vi "User Event AE.vi"(0 "Mode":T3(ring)=enum."Post Event", 1 "Event Name":string, 2 "Event Data":variant, 5 "error in (no error)":errorcluster caption="错误输入（无错误）", 6 "Tag":T1) -> (14 "Event Registration Refnum":T2, 19 "error out":errorcluster caption="错误输出")   [LabVIEW 2013, in "User Event Collection.lvclass"]
uses:
  User Event Collection.lvclass
  <resource>/importtools/Common/Event/Data Type/Event Registeration Refnum.ctl
  Method/Tag.ctl
  <resource>/importtools/Common/Event/NISAST Event.lvclass
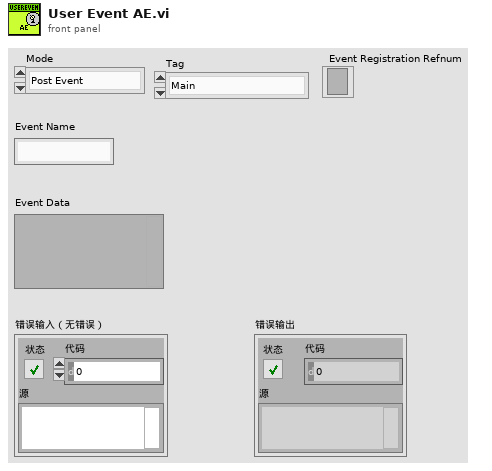
[diagram p1: front panel]
types:
  T1 = typedef "User Event Collection.lvclass/Tag.ctl" = enum16{"Main", "UI"}
  T2 = typedef "NISAST Event.lvclass/Event Registeration Refnum.ctl" = refnum<event-registration>
  T3 = enum16{"Init", "Post Event", "Destroy", "Reg Ref"}
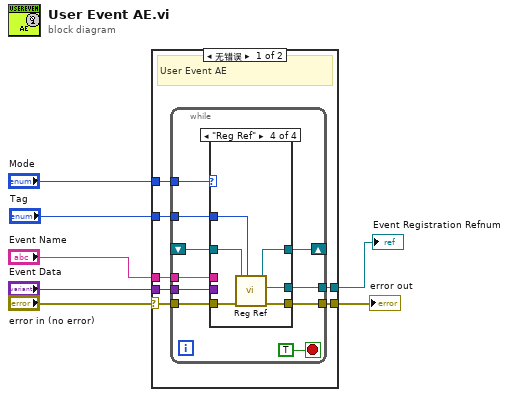
[diagram p0: block diagram]
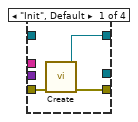
[diagram p2: hidden frame]
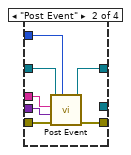
[diagram p3: hidden frame]
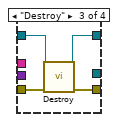
[diagram p4: hidden frame]
diagram:
  n1 = case shown="无错误" "error in (no error)" {
    selector: "error in (no error)" -> [w13 w45]
    tunnel: "Mode" -> [w14 _]
    tunnel: [w12 w45] -> w5
    tunnel: "Event Name" -> [w11 _]
    tunnel: "Event Data" -> [w10 _]
    tunnel: [w9 _] -> w2
    tunnel: "Tag" -> [w8 _]
    frame No Error {
      # "User Event AE"
      n2 = while {
        tunnel: w14 -> [w24]
        shift-right: [w20] -> _
        shift-left: _ -> [w23]
        tunnel: w13 -> [w22]
        tunnel: [w21] -> w12
        tunnel: w11 -> [w19]
        tunnel: w10 -> [w18]
        tunnel: [w17] -> w9
        tunnel: w8 -> [w15]
        stop <- TRUE stop-if-true
        n3 = case shown="\"Reg Ref\"" w24 {
          tunnel: w23 -> [_ w34 w38 w44]
          tunnel: w22 -> [w27 w30 w37 w43]
          tunnel: [w26 w29 w35 w42] -> w21
          tunnel: [w25 w33 w36 w41] -> w20
          tunnel: w19 -> [_ w32 _ _]
          tunnel: w18 -> [_ w31 _ _]
          tunnel: [_ _ _ w40] -> w17
          tunnel: w15 -> [_ w28 _ w39]
          frame "Init", Default {
            n4 = call "Create.vi"("error in (no error)"=w27) -> ("error out"=w26:errorcluster, "User Event Collection 输出"=w25:refnum<class "User Event Collection.lvclass">)  [unwired: 9 in]
          }
          frame "Post Event" {
            n5 = call "Post Event.vi"("Tag"=w28, "error in (no error)"=w30, "Event Data"=w31, "Event Name"=w32, "User Event Collection 输入"=w34) -> ("error out"=w29:errorcluster, "User Event Collection 输出"=w33:refnum<class "User Event Collection.lvclass">)  [unwired: 5 in]
          }
          frame "Destroy" {
            n6 = call "Destroy.vi"("error in (no error)"=w37, "User Event Collection 输入"=w38) -> ("error out"=w35:errorcluster, "User Event Collection 输出"=w36:refnum<class "User Event Collection.lvclass">)  [unwired: 8 in]
          }
          frame "Reg Ref" {
            n7 = call "Reg Ref.vi"("Tag"=w39, "error in (no error)"=w43, "User Event Collection 输入"=w44) -> ("error out"=w42:errorcluster, "Event Registration Refnum"=w40:T2, "User Event Collection 输出"=w41:refnum<class "User Event Collection.lvclass">)  [unwired: 6 in]
          }
        }
      }
    }
    frame Error {
    }
  }
  "error out" <- w5
  "Event Registration Refnum" <- w2
